vi "Save Data.vi"(7 "Detector Manager":refnum<class "Detector Manager.lvclass">, 8 "error in (no error)":errorcluster, 11 "Father Of All Detectors in":refnum<class "Father Of All Detectors.lvclass">) -> (0 "error out":errorcluster, 2 "Data out":variant, 3 "Father Of All Detectors out":refnum<class "Father Of All Detectors.lvclass">)   [LabVIEW 2026, in "TALOS.lvlib" / "Father Of All Detectors.lvlib" / "Father Of All Detectors.lvclass"]
doc: "To optionally send the data also to the DAQ, output if from this VI together setting True the \"Send Data to DAQ?\" output."
uses:
  Father Of All Detectors.lvclass
  Internal uServices/System uServices/Detector Manager/Detector Manager/Detector Manager.lvclass
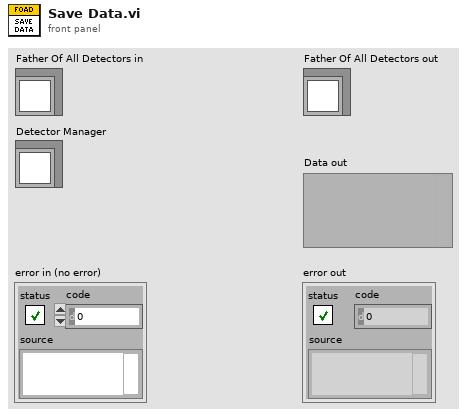
[diagram p1: front panel]
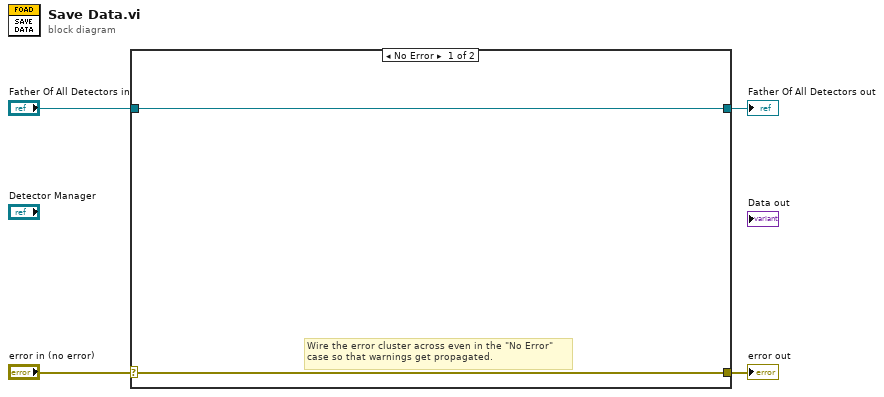
[diagram p0: block diagram]
diagram:
  n1 = case shown="No Error" "error in (no error)" {
    selector: "error in (no error)" -> [w5 w8]
    tunnel: [w5 w8] -> w3
    tunnel: [w6 w7] -> w1
    tunnel: "Father Of All Detectors in" -> [w6 w7]
    frame No Error {
      # "Wire the error cluster across even in the \"No Error\"\ncase so that warnings get propagated."
    }
    frame Error {
    }
  }
  "error out" <- w3
  "Father Of All Detectors out" <- w1
